vi "Setup Hardware Settings.vi"(8 "error in (no error)":errorcluster, 10 "Model in":refnum<class "Model.lvclass">, 11 "Boot Loader in":refnum<class "Boot Loader.lvclass">) -> (0 "error out":errorcluster, 2 "Model out":refnum<class "Model.lvclass">, 3 "Boot Loader out":refnum<class "Boot Loader.lvclass">)   [LabVIEW 2015, in "Boot Loader.lvclass"]
uses:
  Boot Loader.lvclass
  Model/Model.lvclass
  Model/Model.lvclass/Model.ctl
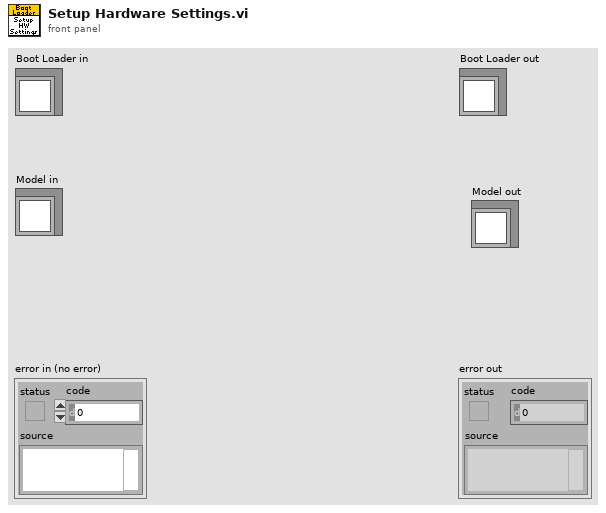
[diagram p1: front panel]
types:
  T1 = typedef "FAMT Typedefs.lvlib/Hardware Settings.ctl" = cluster{"Actuator Types":T2, "Cylinder Types":T3}
  T2 = typedef "FAMT Typedefs.lvlib/Actuator Types.ctl" = enum16{"Single", "Dual"}
  T3 = typedef "FAMT Typedefs.lvlib/Cylinder Types.ctl" = enum16{"PSV Open", "PSV Closed", "TV Open", "TV Closed", "Closed"}
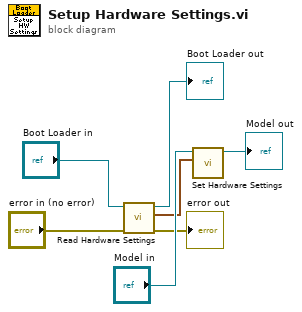
[diagram p0: block diagram]
diagram:
  n1 = call "Read Hardware Settings.vi"("error in (no error)"="error in (no error)", "Boot Loader in"="Boot Loader in") -> ("error out"=→"error out":errorcluster, "Hardware Settings"=w1:T1, "Boot Loader out"=→"Boot Loader out":refnum<class "Boot Loader.lvclass">)  [unwired: 7 in]
  n2 = call "Set Hardware Settings.vi"("Hardware Settings"=w1, "Model in"="Model in") -> ("Model out"=→"Model out":refnum<class "Model.lvclass">)  [unwired: 9 in]
